vi "Battleships_Simulation.vi"() -> ()   [LabVIEW 2015]
doc: "Battleships Simulation VI, European CLA Summit 2017.\n\nUse this VI to help create and test your algorithm VI.\n\nReplace the code of the \"Your code here VI\" with your algorithm for beating the game. Do not change the controls and indicators of this VI and do not modify the connector pane.\n\n- Goal is to win the game by sinking all ships with the least shots possible.\n- Map size is 10x10 squares.\n- Ship sizes are 2, 3, 3, 4, & 5 squares, placed in horizontal or vertical position.\n- Ships are randomly placed each time you execute this VI."
uses:
  TypDefs/Coordinates.ctl
  Classes/Map_class/Map.lvclass
panel:
  out "Grid":u32[][](array[colorbox])
  out "Legend":T1
  out "Last shot fired":T2
  in  "Speed":u32(slide)=500 scale=0.0..1000.0
  out "Statistics":string
  in  "Stop":bool
  # "Battleships Simulation VI\nEuropean CLA Summit 2017"
  # "0"
  # "1"
  # "2"
  # "3"
  # "4"
  # "5"
  # "6"
  # "7"
  # "8"
  # "9"
  # "0"
  # "1"
  # "2"
  # "3"
  # "4"
  # "5"
  # "6"
  # "7"
  # "8"
  # "9"
  # "Slow"
  # "Fast"
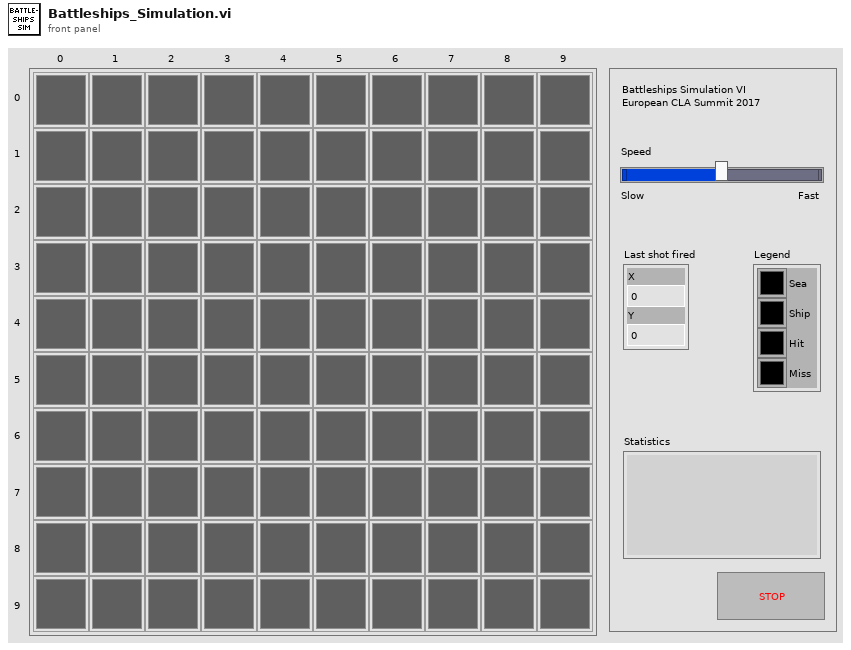
[diagram p1: front panel]
types:
  T1 = cluster{"Sea":u32, "Ship":u32, "Hit":u32, "Miss":u32}
  T2 = typedef "Coordinates.ctl" = cluster{"X":i32, "Y":i32}
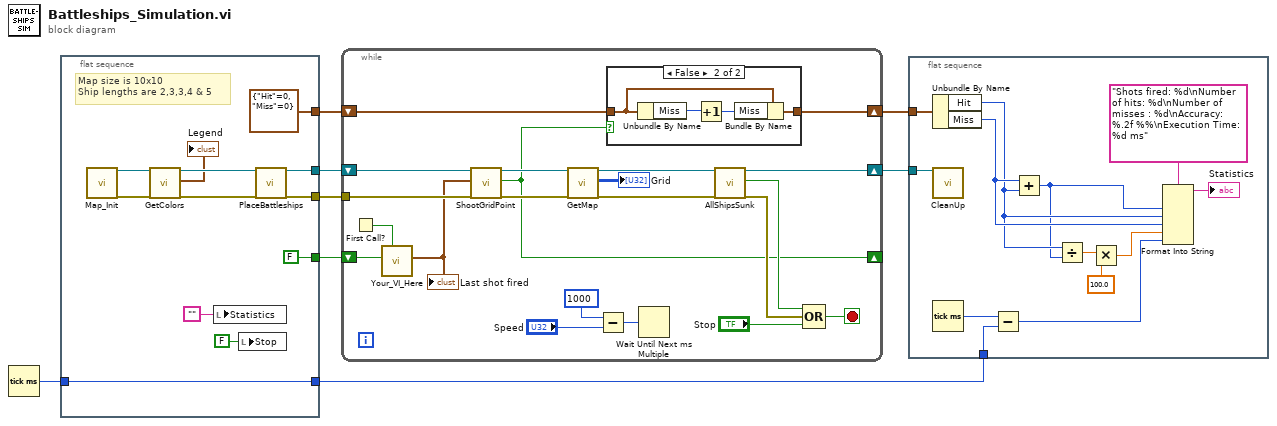
[diagram p0: block diagram]
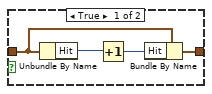
[diagram p2: hidden frame]
diagram:
  n1 = Tick Count (ms)() -> (millisecond timer value=w1:u32)
  n2 = flat-sequence {
    tunnel: [w20] -> w8
    tunnel: [w19] -> w7
    tunnel: [FALSE] -> w5
    tunnel: [cluster{"Hit":i32, "Miss":i32} {"Hit"=0, "Miss"=0}] -> w4
    tunnel: [w9] -> w2
    tunnel: w1 -> [w9]
    frame #0 {
      # "Map size is 10x10\nShip lengths are 2,3,3,4 & 5"
      n3 = call "Map_Init.vi"() -> ("object out"=w14:refnum<class "Map.lvclass">, "error out"=w11:errorcluster)  [unwired: 18 in]
      n4 = call-dynamic "GetColors.vi"("object in"=w14, "error in (no error)"=w11) -> ("object out"=w13:refnum<class "Map.lvclass">, "Colors"=→"Legend":T1, "error out"=w12:errorcluster)  [unwired: 15 in]
      n5 = local write "Statistics"("") -> ()
      n6 = local write "Stop"(FALSE ("stop")) -> ()
      n7 = call-dynamic "PlaceBattleships.vi"("object in"=w13, "error in (no error)"=w12) -> ("object out"=w19:refnum<class "Map.lvclass">, "error out"=w20:errorcluster)  [unwired: 15 in, 1 out]
    }
  }
  n8 = while {
    shift-right: [w38] -> w6
    shift-left: w7 -> [w41]
    tunnel: w8 -> [w37]
    shift-right: [w23] -> _
    shift-left: w5 -> [w30]
    shift-right: [w24] -> w3
    shift-left: w4 -> [w25]
    stop <- w34 stop-if-true
    n9 = First Call?() -> (First Call?: T/F=w22:bool)
    n10 = call "Your_VI_Here.vi"("Reset"=w22, "Hit?"=w30) -> ("Shot\nCoordinates"=w21:T2)  [unwired: 9 in]
    "Last shot fired" <- w21
    n11 = call-dynamic "ShootGridPoint.vi"("object in"=w41, "GridPoint"=w21, "error in (no error)"=w37) -> ("object out"=w40:refnum<class "Map.lvclass">, "Hit?"=w23:bool, "error out"=w36:errorcluster)  [unwired: 13 in, 1 out]
    n12 = call-dynamic "GetMap.vi"("object in"=w40, "error in (no error)"=w36) -> ("object out"=w39:refnum<class "Map.lvclass">, "Grid"=→"Grid":u32[][], "error out"=w35:errorcluster)  [unwired: 15 in]
    n13 = Subtract(x=u32 1000 ("y"), y="Speed") -> (x-y=w26:u32)
    n14 = case shown="False" w23 {
      tunnel: w25 -> [w45 w49]
      tunnel: [w44 w48] -> w24
      frame True {
        n15 = Unbundle By Name(w45) -> ("Hit"=w42:i32)
        n16 = Increment(x=w42) -> (x+1=w43:i32)
        n17 = Bundle By Name(cluster=w45, "Hit"=w43) -> (w44:cluster{"Hit":i32, "Miss":i32})
      }
      frame False {
        n18 = Unbundle By Name(w49) -> ("Miss"=w46:i32)
        n19 = Increment(x=w46) -> (x+1=w47:i32)
        n20 = Bundle By Name(cluster=w49, "Miss"=w47) -> (w48:cluster{"Hit":i32, "Miss":i32})
      }
    }
    n21 = Wait Until Next ms Multiple(millisecond multiple=w26) -> ()  [unwired: 1 out]
    n22 = call-dynamic "AllShipsSunk.vi"("object in"=w39, "error in (no error)"=w35) -> ("object out"=w38:refnum<class "Map.lvclass">, "AllShipsSunk?"=w32:bool, "error out"=w33:errorcluster)  [unwired: 15 in]
    n23 = Compound Arithmetic op=OR(w32, w33, "Stop") -> (w34:bool)
  }
  n24 = flat-sequence {
    tunnel: w6 -> [w62]
    tunnel: w3 -> [w61]
    tunnel: w2 -> [w58]
    frame #0 {
      n25 = Unbundle By Name(w61) -> ("Hit"=w51:i32, "Miss"=w52:i32)
      n26 = call-dynamic "CleanUp.vi"("object in"=w62) -> ()  [unwired: 17 in, 2 out]
      n27 = Tick Count (ms)() -> (millisecond timer value=w59:u32)
      n28 = Subtract(x=w59, y=w58) -> (x-y=w56:u32)
      n29 = Add(x=w52, y=w51) -> (x+y=w50:i32)
      n30 = Divide(x=w51, y=w50) -> (x/y=w55:dbl)
      n31 = Multiply(x=w55, y=100.0) -> (x*y=w53:dbl)
      n32 = Format Into String(format string="Shots fired: %d\nNumber of hits: %d\nNumber of misses : %d\nAccuracy: %.2f %%\nExecution Time: %d ms", w50, w51, w52, w53, w56) -> (resulting string=→"Statistics":string)  [unwired: 2 in, 1 out]
    }
  }
